vi "WLAN DUT Additional Defaults.vi"(0 "niDTS WLAN DUT in":refnum<class "niDTS WLAN Dut.lvclass">, 11 "error in (no error)":errorcluster) -> (4 "niDTS WLAN DUT out":refnum<class "niDTS WLAN Dut.lvclass">, 15 "error out":errorcluster)   [LabVIEW 2015, in "niDTS WLAN.lvlib" / "niDTS WLAN Dut.lvclass"]
doc: "This allows additional defaults to be set after the primary parameters (Standard, Rate, Bandwidth, Streams) have been set. The base additionally sets FEC Coding (BCC for HT and LDPC for VHT) and 16 symbols to True. This can be overridden by specific DUT controllers to impliment the desired behavior."
uses:
  niDTS WLAN Dut.lvclass
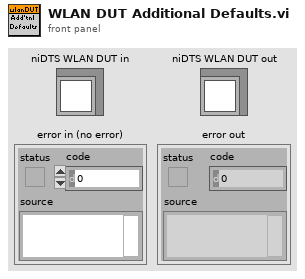
[diagram p1: front panel]
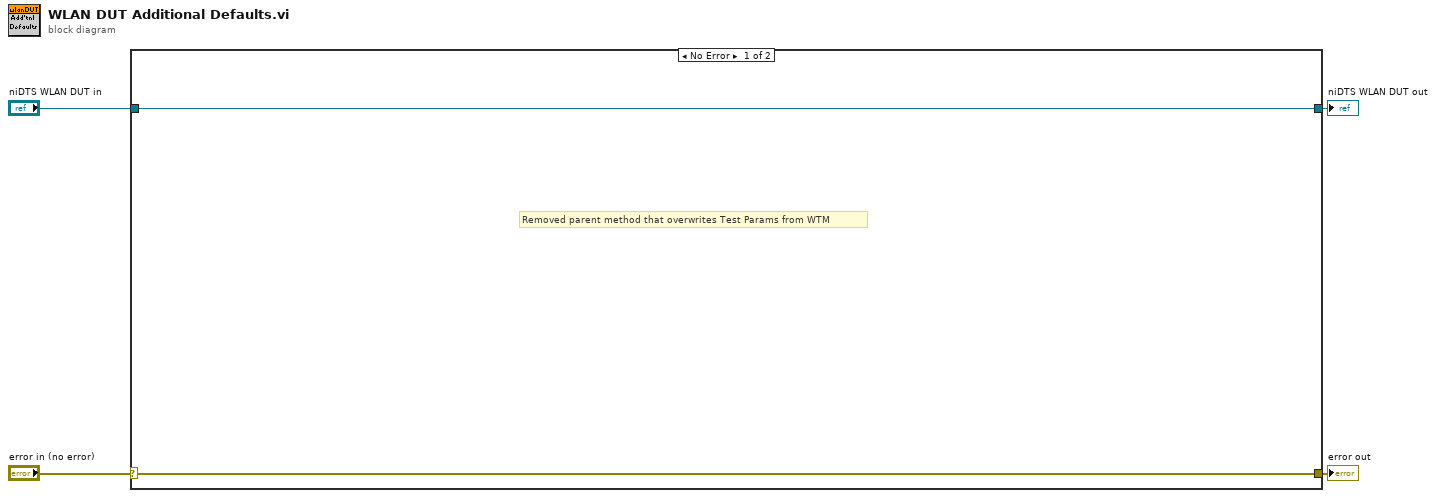
[diagram p0: block diagram]
diagram:
  n1 = case shown="No Error" "error in (no error)" {
    selector: "error in (no error)" -> [w6 w8]
    tunnel: [w6 w8] -> w3
    tunnel: [w5 w7] -> w1
    tunnel: "niDTS WLAN DUT in" -> [w5 w7]
    frame No Error {
      # "Removed parent method that overwrites Test Params from WTM"
    }
    frame Error {
    }
  }
  "error out" <- w3
  "niDTS WLAN DUT out" <- w1
